vi "Get 4 Tables BY WB.vi"(0 "Air Pressure [psia]":dbl, 3 "Wet Bulb Temp [DegF]":dbl) -> (1 "Pressure Z":dbl=53.278814892593125, 4 "WB Z":dbl=nan, 5 "HP Higher WB Psych Table":dbl[][](array[numeric])=[[6500.0, 11.55684946, 0.0, -3.734809203, 0.0, 0.0, 0.0, 14.73657647, 0.0, 0.0], [6500.0, 11.55684946, 5.0, 0.369962485, 0.0, 0.0, 0.0, 14.89687164, 1.2, 0.0], [6500.0, 11.55684946, 10.0, 4.325246632, 0.0, 0.0, 0.0, 15.05716681, 2.4, 0.0], [6500.0, 11.55684946, 15.0, 8.123037731, 0.0, 0.0, 0.0, 15.21746199, 3.6, 0.0], [6500.0, 11.55684946, 20.0, 11.75811873, 0.0, 0.0, 0.0, 15.37775716, 4.8, 0.0], [6500.0, 11.55684946, 25.0, 15.2280745, 0.0, 0.0, 0.0, 15.53805233, 6.0, 0.0], [6500.0, 11.55684946, 30.0, 18.53315425, 0.0, 0.0, 0.0, 15.69834751, 7.2, 0.0], [6500.0, 11.55684946, 35.0, 21.67592924, 0.0, 0.0, 0.0, 15.85864268, 8.4, 0.0], [6500.0, 11.55684946, 40.0, 24.66089526, 0.0, 0.0, 0.0, 16.01893785, 9.6, 0.0], [6500.0, 11.55684946, 45.0, 27.49399256, 0.0, 0.0, 0.0, 16.17923303, 10.8, 0.0], [6500.0, 11.55684946, 50.0, 30.18218136, 0.0, 0.0, 0.0, 16.3395282, 12.0, 0.0], [6500.0, 11.55684946, 55.0, 32.77874534, 0.0, 0.0, 0.0, 16.49982337, 13.2, 0.0], [6500.0, 11.55684946, 60.0, 35.36738433, 0.0, 0.0, 0.0, 16.66011855, 14.4, 0.0], [6500.0, 11.55684946, 65.0, 37.84423533, 0.0, 0.0, 0.0, 16.82041372, 15.6, 0.0], [6500.0, 11.55684946, 70.0, 40.21526739, 0.0, 0.0, 0.0, 16.98070889, 16.8, 0.0], [6500.0, 11.55684946, 75.0, 42.48635581, 0.0, 0.0, 0.0, 17.14100407, 18.0, 0.0], [6500.0, 11.55684946, 80.0, 44.66320929, 0.0, 0.0, 0.0, 17.30129924, 19.2, 0.0], [6500.0, 11.55684946, 85.0, 46.75131137, 0.0, 0.0, 0.0, 17.46159441, 20.4, 0.0], [6500.0, 11.55684946, 90.0, 48.75588828, 0.0, 0.0, 0.0, 17.62188959, 21.6, 0.0], [6500.0, 11.55684946, 95.0, 50.68188865, 0.0, 0.0, 0.0, 17.78218476, 22.8, 0.0], [6500.0, 11.55684946, 100.0, 52.53397522, 0.0, 0.0, 0.0, 17.94247993, 24.0, 0.0], [6500.0, 11.55684946, 105.0, 54.31652083, 0.0, 0.0, 0.0, 18.10277511, 25.2, 0.0], [6500.0, 11.55684946, 110.0, 56.03362328, 0.0, 0.0, 0.0, 18.26307028, 26.4, 0.0], [6500.0, 11.55684946, 115.0, 57.68910488, 0.0, 0.0, 0.0, 18.42336545, 27.6, 0.0], [6500.0, 11.55684946, 120.0, 59.28653031, 0.0, 0.0, 0.0, 18.58366063, 28.8, 0.0]], 6 "HP Lower WB Psych Table":dbl[][](array[numeric])=[[6500.0, 11.55684946, 0.0, -3.734809203, 0.0, 0.0, 0.0, 14.73657647, 0.0, 0.0], [6500.0, 11.55684946, 5.0, 0.369962485, 0.0, 0.0, 0.0, 14.89687164, 1.2, 0.0], [6500.0, 11.55684946, 10.0, 4.325246632, 0.0, 0.0, 0.0, 15.05716681, 2.4, 0.0], [6500.0, 11.55684946, 15.0, 8.123037731, 0.0, 0.0, 0.0, 15.21746199, 3.6, 0.0], [6500.0, 11.55684946, 20.0, 11.75811873, 0.0, 0.0, 0.0, 15.37775716, 4.8, 0.0], [6500.0, 11.55684946, 25.0, 15.2280745, 0.0, 0.0, 0.0, 15.53805233, 6.0, 0.0], [6500.0, 11.55684946, 30.0, 18.53315425, 0.0, 0.0, 0.0, 15.69834751, 7.2, 0.0], [6500.0, 11.55684946, 35.0, 21.67592924, 0.0, 0.0, 0.0, 15.85864268, 8.4, 0.0], [6500.0, 11.55684946, 40.0, 24.66089526, 0.0, 0.0, 0.0, 16.01893785, 9.6, 0.0], [6500.0, 11.55684946, 45.0, 27.49399256, 0.0, 0.0, 0.0, 16.17923303, 10.8, 0.0], [6500.0, 11.55684946, 50.0, 30.18218136, 0.0, 0.0, 0.0, 16.3395282, 12.0, 0.0], [6500.0, 11.55684946, 55.0, 32.77874534, 0.0, 0.0, 0.0, 16.49982337, 13.2, 0.0], [6500.0, 11.55684946, 60.0, 35.36738433, 0.0, 0.0, 0.0, 16.66011855, 14.4, 0.0], [6500.0, 11.55684946, 65.0, 37.84423533, 0.0, 0.0, 0.0, 16.82041372, 15.6, 0.0], [6500.0, 11.55684946, 70.0, 40.21526739, 0.0, 0.0, 0.0, 16.98070889, 16.8, 0.0], [6500.0, 11.55684946, 75.0, 42.48635581, 0.0, 0.0, 0.0, 17.14100407, 18.0, 0.0], [6500.0, 11.55684946, 80.0, 44.66320929, 0.0, 0.0, 0.0, 17.30129924, 19.2, 0.0], [6500.0, 11.55684946, 85.0, 46.75131137, 0.0, 0.0, 0.0, 17.46159441, 20.4, 0.0], [6500.0, 11.55684946, 90.0, 48.75588828, 0.0, 0.0, 0.0, 17.62188959, 21.6, 0.0], [6500.0, 11.55684946, 95.0, 50.68188865, 0.0, 0.0, 0.0, 17.78218476, 22.8, 0.0], [6500.0, 11.55684946, 100.0, 52.53397522, 0.0, 0.0, 0.0, 17.94247993, 24.0, 0.0], [6500.0, 11.55684946, 105.0, 54.31652083, 0.0, 0.0, 0.0, 18.10277511, 25.2, 0.0], [6500.0, 11.55684946, 110.0, 56.03362328, 0.0, 0.0, 0.0, 18.26307028, 26.4, 0.0], [6500.0, 11.55684946, 115.0, 57.68910488, 0.0, 0.0, 0.0, 18.42336545, 27.6, 0.0], [6500.0, 11.55684946, 120.0, 59.28653031, 0.0, 0.0, 0.0, 18.58366063, 28.8, 0.0]], 7 "LP Higher WB Psych Table":dbl[][](array[numeric])=[[7000.0, 11.3399368, 0.0, -3.79438535, 0.0, 0.0, 0.0, 15.01846076, 0.0, 0.0], [7000.0, 11.3399368, 5.0, 0.298673776, 0.0, 0.0, 0.0, 15.1818221, 1.2, 0.0], [7000.0, 11.3399368, 10.0, 4.241216923, 0.0, 0.0, 0.0, 15.34518343, 2.4, 0.0], [7000.0, 11.3399368, 15.0, 8.025427492, 0.0, 0.0, 0.0, 15.50854476, 3.6, 0.0], [7000.0, 11.3399368, 20.0, 11.64630617, 0.0, 0.0, 0.0, 15.67190609, 4.8, 0.0], [7000.0, 11.3399368, 25.0, 15.10166504, 0.0, 0.0, 0.0, 15.83526743, 6.0, 0.0], [7000.0, 11.3399368, 30.0, 18.39197072, 0.0, 0.0, 0.0, 15.99862876, 7.2, 0.0], [7000.0, 11.3399368, 35.0, 21.52000084, 0.0, 0.0, 0.0, 16.16199009, 8.4, 0.0], [7000.0, 11.3399368, 40.0, 24.49041192, 0.0, 0.0, 0.0, 16.32535143, 9.6, 0.0], [7000.0, 11.3399368, 45.0, 27.30928225, 0.0, 0.0, 0.0, 16.48871276, 10.8, 0.0], [7000.0, 11.3399368, 50.0, 29.98367427, 0.0, 0.0, 0.0, 16.65207409, 12.0, 0.0], [7000.0, 11.3399368, 55.0, 32.55356012, 0.0, 0.0, 0.0, 16.81543542, 13.2, 0.0], [7000.0, 11.3399368, 60.0, 35.12844084, 0.0, 0.0, 0.0, 16.97879676, 14.4, 0.0], [7000.0, 11.3399368, 65.0, 37.59196462, 0.0, 0.0, 0.0, 17.14215809, 15.6, 0.0], [7000.0, 11.3399368, 70.0, 39.95012443, 0.0, 0.0, 0.0, 17.30551942, 16.8, 0.0], [7000.0, 11.3399368, 75.0, 42.20880771, 0.0, 0.0, 0.0, 17.46888075, 18.0, 0.0], [7000.0, 11.3399368, 80.0, 44.37372685, 0.0, 0.0, 0.0, 17.63224209, 19.2, 0.0], [7000.0, 11.3399368, 85.0, 46.45036161, 0.0, 0.0, 0.0, 17.79560342, 20.4, 0.0], [7000.0, 11.3399368, 90.0, 48.44392936, 0.0, 0.0, 0.0, 17.95896475, 21.6, 0.0], [7000.0, 11.3399368, 95.0, 50.35936607, 0.0, 0.0, 0.0, 18.12232609, 22.8, 0.0], [7000.0, 11.3399368, 100.0, 52.20131935, 0.0, 0.0, 0.0, 18.28568742, 24.0, 0.0], [7000.0, 11.3399368, 105.0, 53.97414441, 0.0, 0.0, 0.0, 18.44904875, 25.2, 0.0], [7000.0, 11.3399368, 110.0, 55.68192183, 0.0, 0.0, 0.0, 18.61241008, 26.4, 0.0], [7000.0, 11.3399368, 115.0, 57.32845529, 0.0, 0.0, 0.0, 18.77577142, 27.6, 0.0], [7000.0, 11.3399368, 120.0, 58.91729107, 0.0, 0.0, 0.0, 18.93913275, 28.8, 0.0]], 8 "LP Lower WB Psych Table":dbl[][](array[numeric])=[[7000.0, 11.3399368, 0.0, -3.79438535, 0.0, 0.0, 0.0, 15.01846076, 0.0, 0.0], [7000.0, 11.3399368, 5.0, 0.298673776, 0.0, 0.0, 0.0, 15.1818221, 1.2, 0.0], [7000.0, 11.3399368, 10.0, 4.241216923, 0.0, 0.0, 0.0, 15.34518343, 2.4, 0.0], [7000.0, 11.3399368, 15.0, 8.025427492, 0.0, 0.0, 0.0, 15.50854476, 3.6, 0.0], [7000.0, 11.3399368, 20.0, 11.64630617, 0.0, 0.0, 0.0, 15.67190609, 4.8, 0.0], [7000.0, 11.3399368, 25.0, 15.10166504, 0.0, 0.0, 0.0, 15.83526743, 6.0, 0.0], [7000.0, 11.3399368, 30.0, 18.39197072, 0.0, 0.0, 0.0, 15.99862876, 7.2, 0.0], [7000.0, 11.3399368, 35.0, 21.52000084, 0.0, 0.0, 0.0, 16.16199009, 8.4, 0.0], [7000.0, 11.3399368, 40.0, 24.49041192, 0.0, 0.0, 0.0, 16.32535143, 9.6, 0.0], [7000.0, 11.3399368, 45.0, 27.30928225, 0.0, 0.0, 0.0, 16.48871276, 10.8, 0.0], [7000.0, 11.3399368, 50.0, 29.98367427, 0.0, 0.0, 0.0, 16.65207409, 12.0, 0.0], [7000.0, 11.3399368, 55.0, 32.55356012, 0.0, 0.0, 0.0, 16.81543542, 13.2, 0.0], [7000.0, 11.3399368, 60.0, 35.12844084, 0.0, 0.0, 0.0, 16.97879676, 14.4, 0.0], [7000.0, 11.3399368, 65.0, 37.59196462, 0.0, 0.0, 0.0, 17.14215809, 15.6, 0.0], [7000.0, 11.3399368, 70.0, 39.95012443, 0.0, 0.0, 0.0, 17.30551942, 16.8, 0.0], [7000.0, 11.3399368, 75.0, 42.20880771, 0.0, 0.0, 0.0, 17.46888075, 18.0, 0.0], [7000.0, 11.3399368, 80.0, 44.37372685, 0.0, 0.0, 0.0, 17.63224209, 19.2, 0.0], [7000.0, 11.3399368, 85.0, 46.45036161, 0.0, 0.0, 0.0, 17.79560342, 20.4, 0.0], [7000.0, 11.3399368, 90.0, 48.44392936, 0.0, 0.0, 0.0, 17.95896475, 21.6, 0.0], [7000.0, 11.3399368, 95.0, 50.35936607, 0.0, 0.0, 0.0, 18.12232609, 22.8, 0.0], [7000.0, 11.3399368, 100.0, 52.20131935, 0.0, 0.0, 0.0, 18.28568742, 24.0, 0.0], [7000.0, 11.3399368, 105.0, 53.97414441, 0.0, 0.0, 0.0, 18.44904875, 25.2, 0.0], [7000.0, 11.3399368, 110.0, 55.68192183, 0.0, 0.0, 0.0, 18.61241008, 26.4, 0.0], [7000.0, 11.3399368, 115.0, 57.32845529, 0.0, 0.0, 0.0, 18.77577142, 27.6, 0.0], [7000.0, 11.3399368, 120.0, 58.91729107, 0.0, 0.0, 0.0, 18.93913275, 28.8, 0.0]])   [LabVIEW 2020]
panel:
  in  "WB Array":dbl[](array[numeric])=[0.0, 5.0, 10.0, 15.0, 20.0, 25.0, 30.0, 35.0, 40.0, 45.0, 50.0, 55.0, 60.0, 65.0, 70.0, 75.0, 80.0, 85.0, 90.0, 95.0, 100.0, 105.0, 110.0, 115.0, 120.0]
  in  "Pressure Array":dbl[](array[numeric])=[15.51026974, 15.23488864, 14.96348006, 14.696, 14.43240481, 14.17265118, 13.91669613, 13.66449702, 13.41601153, 13.17119769, 12.93001384, 12.69241866, 12.45837117, 12.22783068, 12.00075687, 11.77710969, 11.55684946, 11.3399368]
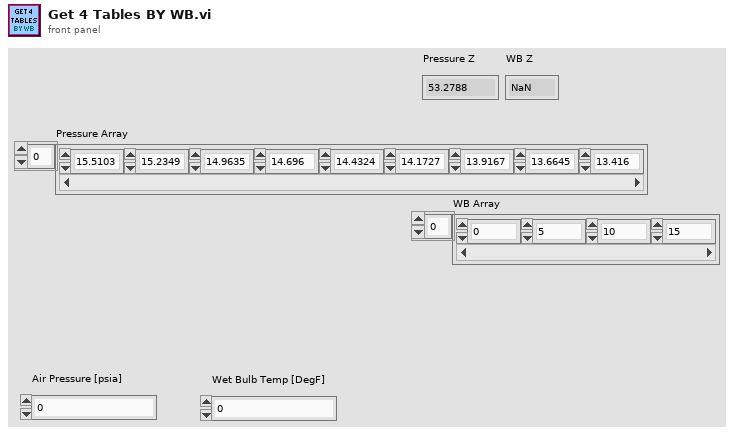
[diagram p1: front panel]
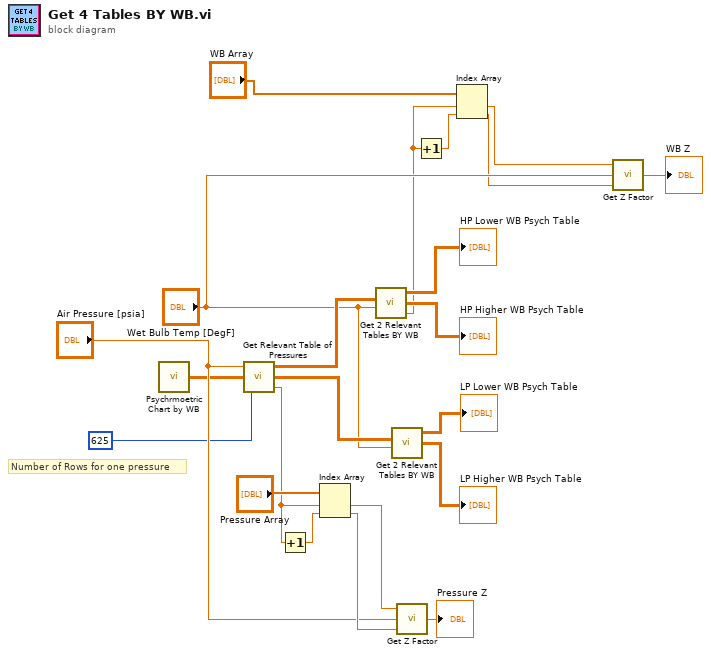
[diagram p0: block diagram]
diagram:
  # "Number of Rows for one pressure"
  n1 = call "Psychrmoetric Chart by WB.vi"() -> ("Psych Chart by WB"=w1:dbl[][])
  n2 = call "Get Relevant Table of Pressures.vi"("Length of List for 1 Pressure"=625 ("Length of List for a Single Pressure"), "Psych Table"=w1, "Air Pressure [psia]"="Air Pressure [psia]") -> ("Pressure Index"=w13:dbl, "Lower Pressure Psych Table"=w19:dbl[][], "Higher Pressure Psych Table"=w22:dbl[][])
  n3 = Increment(x=w13) -> (x+1=w12:dbl)
  n4 = Index Array(array="Pressure Array", index #1=w13, index #2=w12) -> (element #1=w11:dbl, element #2=w10:dbl)
  n5 = call "Get 2 Relevant Tables BY WB.vi"("Psych Table"=w22, "Wet Bulb Temp [DegF]"="Wet Bulb Temp [DegF]") -> ("Lower WB Psych Table"=→"HP Lower WB Psych Table":dbl[][], "Higher WB Psych Table"=→"HP Higher WB Psych Table":dbl[][], "WB Index"=w8:dbl)  [unwired: 4 in]
  n6 = call "Get 2 Relevant Tables BY WB.vi"("Psych Table"=w19, "Wet Bulb Temp [DegF]"="Wet Bulb Temp [DegF]") -> ("Lower WB Psych Table"=→"LP Lower WB Psych Table":dbl[][], "Higher WB Psych Table"=→"LP Higher WB Psych Table":dbl[][])  [unwired: 4 in, 1 out]
  n7 = call "Get Z Factor.vi"("X2"=w10, "Xi"="Air Pressure [psia]", "X1"=w11) -> ("Z"=→"Pressure Z":dbl)  [unwired: 2 in]
  n8 = Increment(x=w8) -> (x+1=w9:dbl)
  n9 = Index Array(array="WB Array", index #1=w8, index #2=w9) -> (element #1=w7:dbl, element #2=w6:dbl)
  n10 = call "Get Z Factor.vi"("X2"=w6, "Xi"="Wet Bulb Temp [DegF]", "X1"=w7) -> ("Z"=→"WB Z":dbl)  [unwired: 2 in]
